vi "main_qsm.vi"() -> ()   [LabVIEW 2024]
uses:
  qsm support/queue_state_&_argument (Array).vi
  <vilib>/Utility/error.llb/Error Cluster From Error Code.vi
  qsm support/queue_state_&_argument (Single).vi
  <vilib>/ErrorRing/Error Ring.xnode
panel:
  out "filenames":string[](array[string])
  in  "Run Test 2":bool
  in  "Get csv files data":bool
  in  "Stop Button":bool
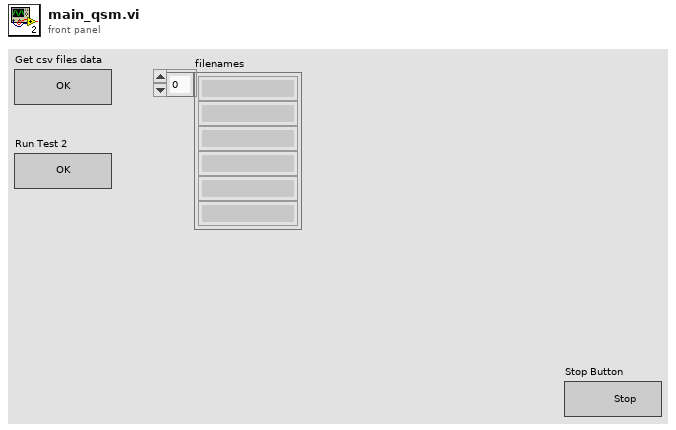
[diagram p1: front panel]
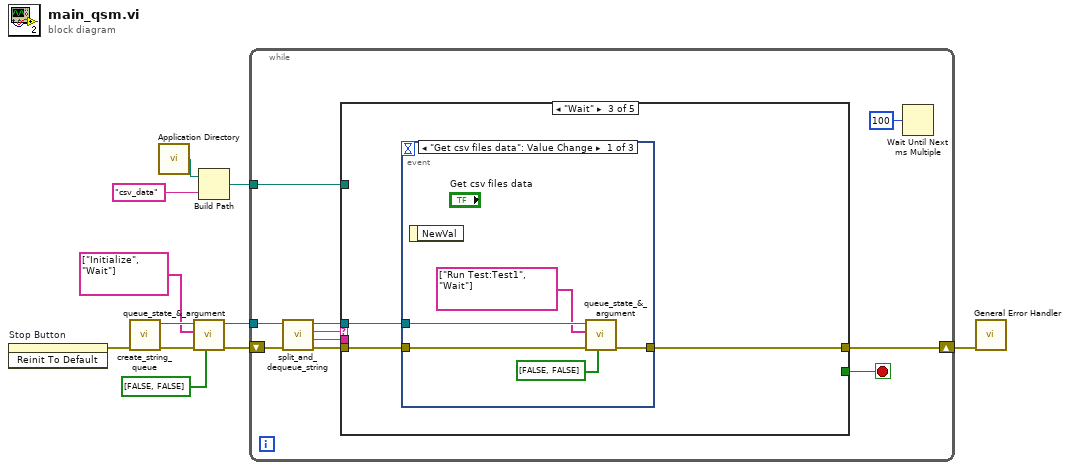
[diagram p0: block diagram]
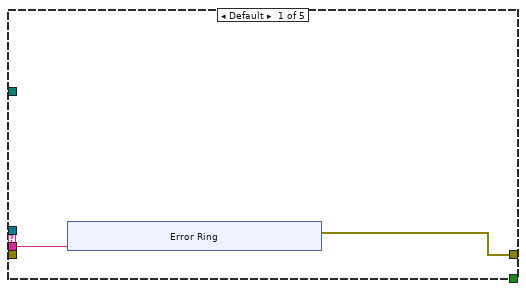
[diagram p2: hidden frame]
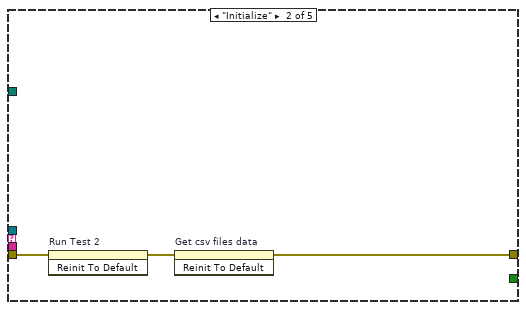
[diagram p3: hidden frame]
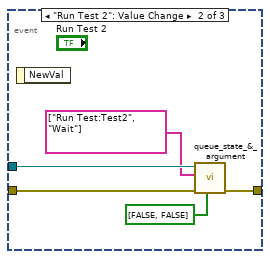
[diagram p4: hidden frame]
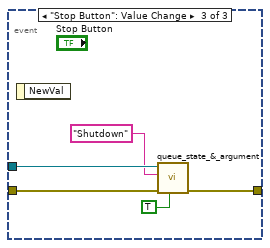
[diagram p5: hidden frame]
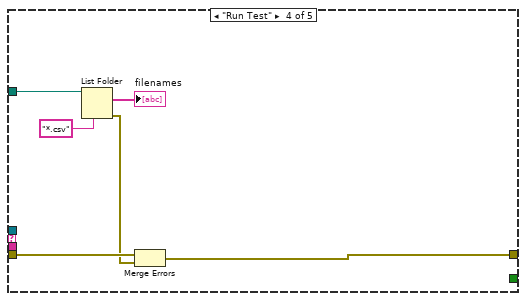
[diagram p6: hidden frame]
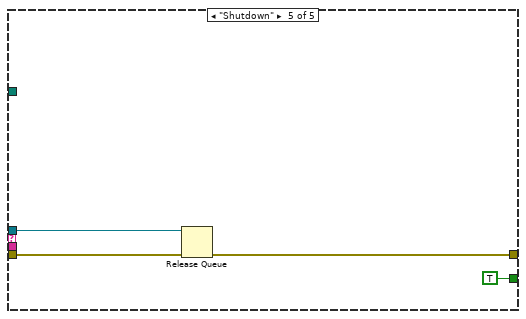
[diagram p7: hidden frame]
diagram:
  n1 = invoke on="Stop Button" class="Bool" method="Reinit To Default"() -> (error out=w10:errorcluster)  [unwired: 3 in, 2 out]
  n2 = call "create_string_queue.vi"("error in (no error)"=w10) -> ("error out"=w8:errorcluster, "Queue out"=w7:refnum<queue>)  [unwired: 9 in]
  n3 = call <vilib>:"Application Directory.vi"() -> ("Application Directory"=w3:path)
  n4 = call-poly "queue_state_&_argument.vi"("Priority? Array"=bool[] [FALSE, FALSE], "error in (no error)"=w8, "state:argument array"=string[] ["Initialize", "Wait"], "Queue in"=w7) -> ("error out"=w9:errorcluster, "Queue out"=w6:refnum<queue>)  [unwired: 6 in]
  n5 = Build Path(base path=w3, name or relative path="csv_data") -> (appended path=w1:path)
  n6 = while {
    shift-right: [w20] -> w11
    shift-left: w9 -> [w14]
    tunnel: w6 -> [w13]
    tunnel: w1 -> [w12]
    stop <- w19 stop-if-true
    n7 = call "split_and_dequeue_string.vi"("error in (no error)"=w14, "Queue in"=w13) -> ("error out"=w17:errorcluster, "argument"=w15:string, "state"=w16:string, "Queue out"=w18:refnum<queue>)  [unwired: 6 in]
    n8 = case shown="\"Wait\"" w16 {
      tunnel: w17 -> [_ w33 w36 w57 w60]
      tunnel: [w22 w31 w35 w54 w58] -> w20
      tunnel: [_ _ _ _ TRUE] -> w19
      tunnel: w18 -> [_ _ w34 _ w59]
      tunnel: w15 -> [w23 _ _ _ _]
      tunnel: w12 -> [_ _ _ w56 _]
      frame Default {
        n9 = xnode "Error Ring"("parameter 0"=w23) -> ("error out"=w22:errorcluster)
      }
      frame "Initialize" {
        n10 = invoke on="Run Test 2" class="Bool" method="Reinit To Default"(error in=w33) -> (error out=w32:errorcluster)  [unwired: 2 in, 2 out]
        n11 = invoke on="Get csv files data" class="Bool" method="Reinit To Default"(error in=w32) -> (error out=w31:errorcluster)  [unwired: 2 in, 2 out]
      }
      frame "Wait" {
        n12 = event shown="[0] \"Get csv files data\": Value Change" {
          selector: _ -> [_ _ _]
          dyn-events: _ -> [_ _ _]
          timeout: _ -> [_ _ _]
          tunnel: w36 -> [w40 w46 w50]
          tunnel: [w39 w45 w51] -> w35
          tunnel: w34 -> [w38 w44 w49]
          event "Get csv files data": Value Change {
            n13 = event-data() -> ()  [unwired: 1 in, 1 out]
            n14 = call-poly "queue_state_&_argument.vi"("Priority? Array"=bool[] [FALSE, FALSE], "error in (no error)"=w40, "state:argument array"=string[] ["Run Test:Test1", "Wait"], "Queue in"=w38) -> ("error out"=w39:errorcluster)  [unwired: 6 in, 1 out]
          }
          event "Run Test 2": Value Change {
            n15 = event-data() -> ()  [unwired: 1 in, 1 out]
            n16 = call-poly "queue_state_&_argument.vi"("Priority? Array"=bool[] [FALSE, FALSE], "error in (no error)"=w46, "state:argument array"=string[] ["Run Test:Test2", "Wait"], "Queue in"=w44) -> ("error out"=w45:errorcluster)  [unwired: 6 in, 1 out]
          }
          event "Stop Button": Value Change {
            n17 = event-data() -> ()  [unwired: 1 in, 1 out]
            n18 = call-poly "queue_state_&_argument.vi"("Priority? (F)"=TRUE, "error in (no error)"=w50, "state:argument"="Shutdown", "Queue in"=w49) -> ("error out"=w51:errorcluster)  [unwired: 6 in, 1 out]
          }
        }
      }
      frame "Run Test" {
        n19 = List Folder(path=w56, pattern="*.csv") -> (filenames=→"filenames":string[], error out=w53:errorcluster)  [unwired: 2 in, 2 out]
        n20 = Merge Errors(w57, w53) -> (w54:errorcluster)
      }
      frame "Shutdown" {
        n21 = Release Queue(queue=w59, error in (no error)=w60) -> (error out=w58:errorcluster)  [unwired: 1 in, 2 out]
      }
    }
    n22 = Wait Until Next ms Multiple(millisecond multiple=u32 100) -> ()  [unwired: 1 out]
  }
  n23 = call <vilib>:"General Error Handler.vi"("error in (no error)"=w11) -> ()  [unwired: 10 in, 5 out]
